vi "Set Peaks In Gate [PIG].vi"(7 "Micropulse # In":i32, 8 "error in (no error)":errorcluster, 10 "# Peaks to report":u16) -> (0 "error out":errorcluster, 5 "Micropulse # Out":i32)   [LabVIEW 2026, in "MicroPulse_Driver.lvlib"]
doc: "Used to define how many peaks are reported in AMP mode 2. The first n-1 plus the largest of the remaining peaks are reported.\n\nParameters:\n<Value> : Integer value n from 1 to 80"
uses:
  MicroPulse_Driver.lvlib
  Private/MP-Registry Action-Enum.ctl
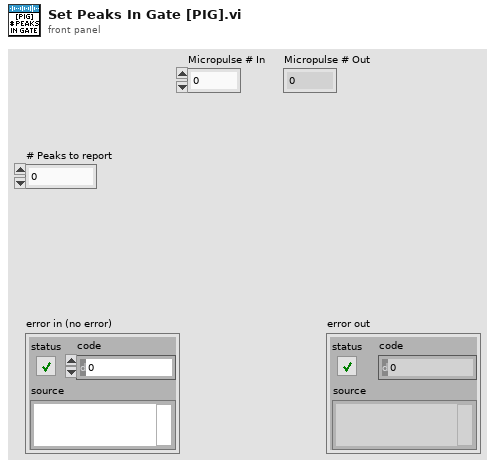
[diagram p1: front panel]
types:
  T1 = typedef "MicroPulse_Driver.lvlib/MP-Registry Action-Enum.ctl" = enum16{"Read", "Add Test", "Add Command", "Add Gate Command", "Add Encoder Command", "Clear Command  List", "Set Registry", "Set System Details", "Set DOF", "Set Velocity", "Disable Asynch Reads", "Enable Asynch Reads", "Add Connection", "Disconnect", "Shutdown"}
  T2 = typedef "Micropulse.lvlib/TCP config.ctl" = cluster{"Connection ID":refnum<k5>, "IP address":string, "host port":u16, "OC timeout":i32, "Read timeout":i32, "Write timeout":i32}
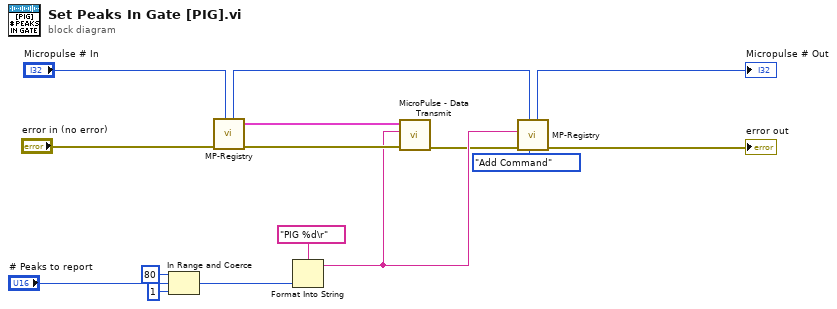
[diagram p0: block diagram]
diagram:
  n1 = In Range and Coerce(upper limit=u16 80, x="# Peaks to report", lower limit=u16 1) -> (coerced(x)=w3:u16)  [unwired: 1 out]
  n2 = call "MP-Registry.vi"("Micropulse # In"="Micropulse # In", "error in (no error)"="error in (no error)") -> ("error out"=w13:errorcluster, "TCP config"=w12:T2, "Micropulse # Out"=w8:i32)  [unwired: 6 in, 1 out]
  n3 = Format Into String(format string="PIG %d\r", w3) -> (resulting string=w11:string)  [unwired: 2 in, 1 out]
  n4 = call "MicroPulse - Data Transmit.vi"("error in (no error)"=w13, "data"=w11, "TCP config"=w12) -> ("error out"=w9:errorcluster)  [unwired: 6 in, 2 out]
  n5 = call "MP-Registry.vi"("Action"=MP-Registry_Action-Enum."Add Command", "Micropulse # In"=w8, "error in (no error)"=w9, "Data in"=w11) -> ("error out"=→"error out":errorcluster, "Micropulse # Out"=→"Micropulse # Out":i32)  [unwired: 4 in, 2 out]
